vi "Main.vi"() -> ()   [LabVIEW 2021]
uses:
  <vilib>/Instr/_visa.llb/VISA Configure Serial Port (Instr).vi
panel:
  in  "Baud":string(combo)="9600"
  in  "Line Ending":string(combo)="0"
  in  "COM Port":refnum<visa-resource-name>="COM6"
  in  "Enter":bool
  in  "CLEAR":bool
  in  "RESTART COMPORT":bool
  in  "Write to Serial":string
  out "Read from Serial":string
  out "Serial_Thread_state":dbl
  out "Serial_Thread_counter":dbl
  out "Save_Timer_Serial_Thread":dbl
  out "LED_2_state":dbl
  out "LED_2_counter":dbl
  out "Save_Timer_LED_2":dbl
  out "LED_2":bool
  out "Display_1_state":dbl
  out "Display_1_counter":dbl
  out "Save_Timer_Display_1":dbl
  out "LED_1_state":dbl
  out "LED_1_counter":dbl
  out "Save_Timer_LED_1":dbl
  out "LED_1":bool
  in  "Button_1":bool
  in  "Button_2":bool
  in  "CLOSE APP":bool
  out "Display_1":dbl
  # "Press ADD or SUB to add/subtract a value of 1 into the Display_1. Buttons are being monitored while 2 LEDs are\nblinking with different periods. This whole system is executed in multitask process. You may notice that LEDs are\nnot affected nor the buttons are affected to each other. No delay at all."
  # "Note:\nDo not Run the program without Device Connected to the Serial Port.\nIf Error occured because nothing is connected to the comport, just click Continue."
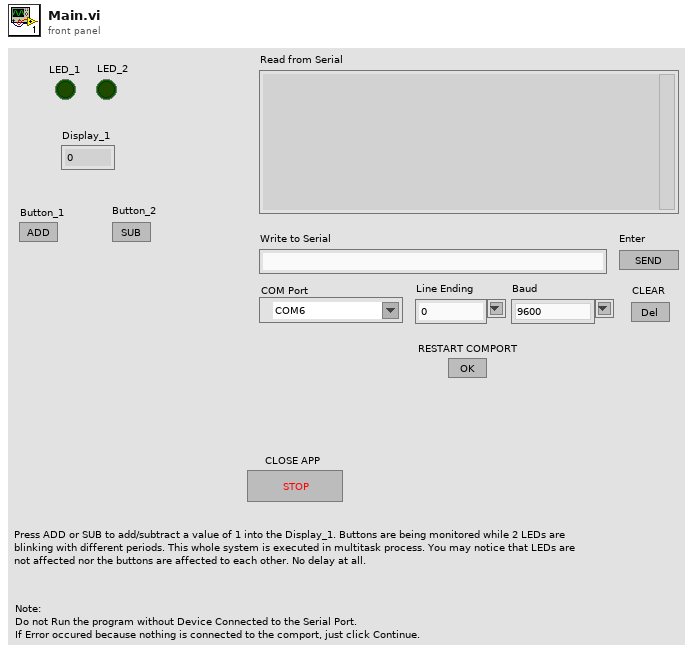
[diagram p1: front panel]
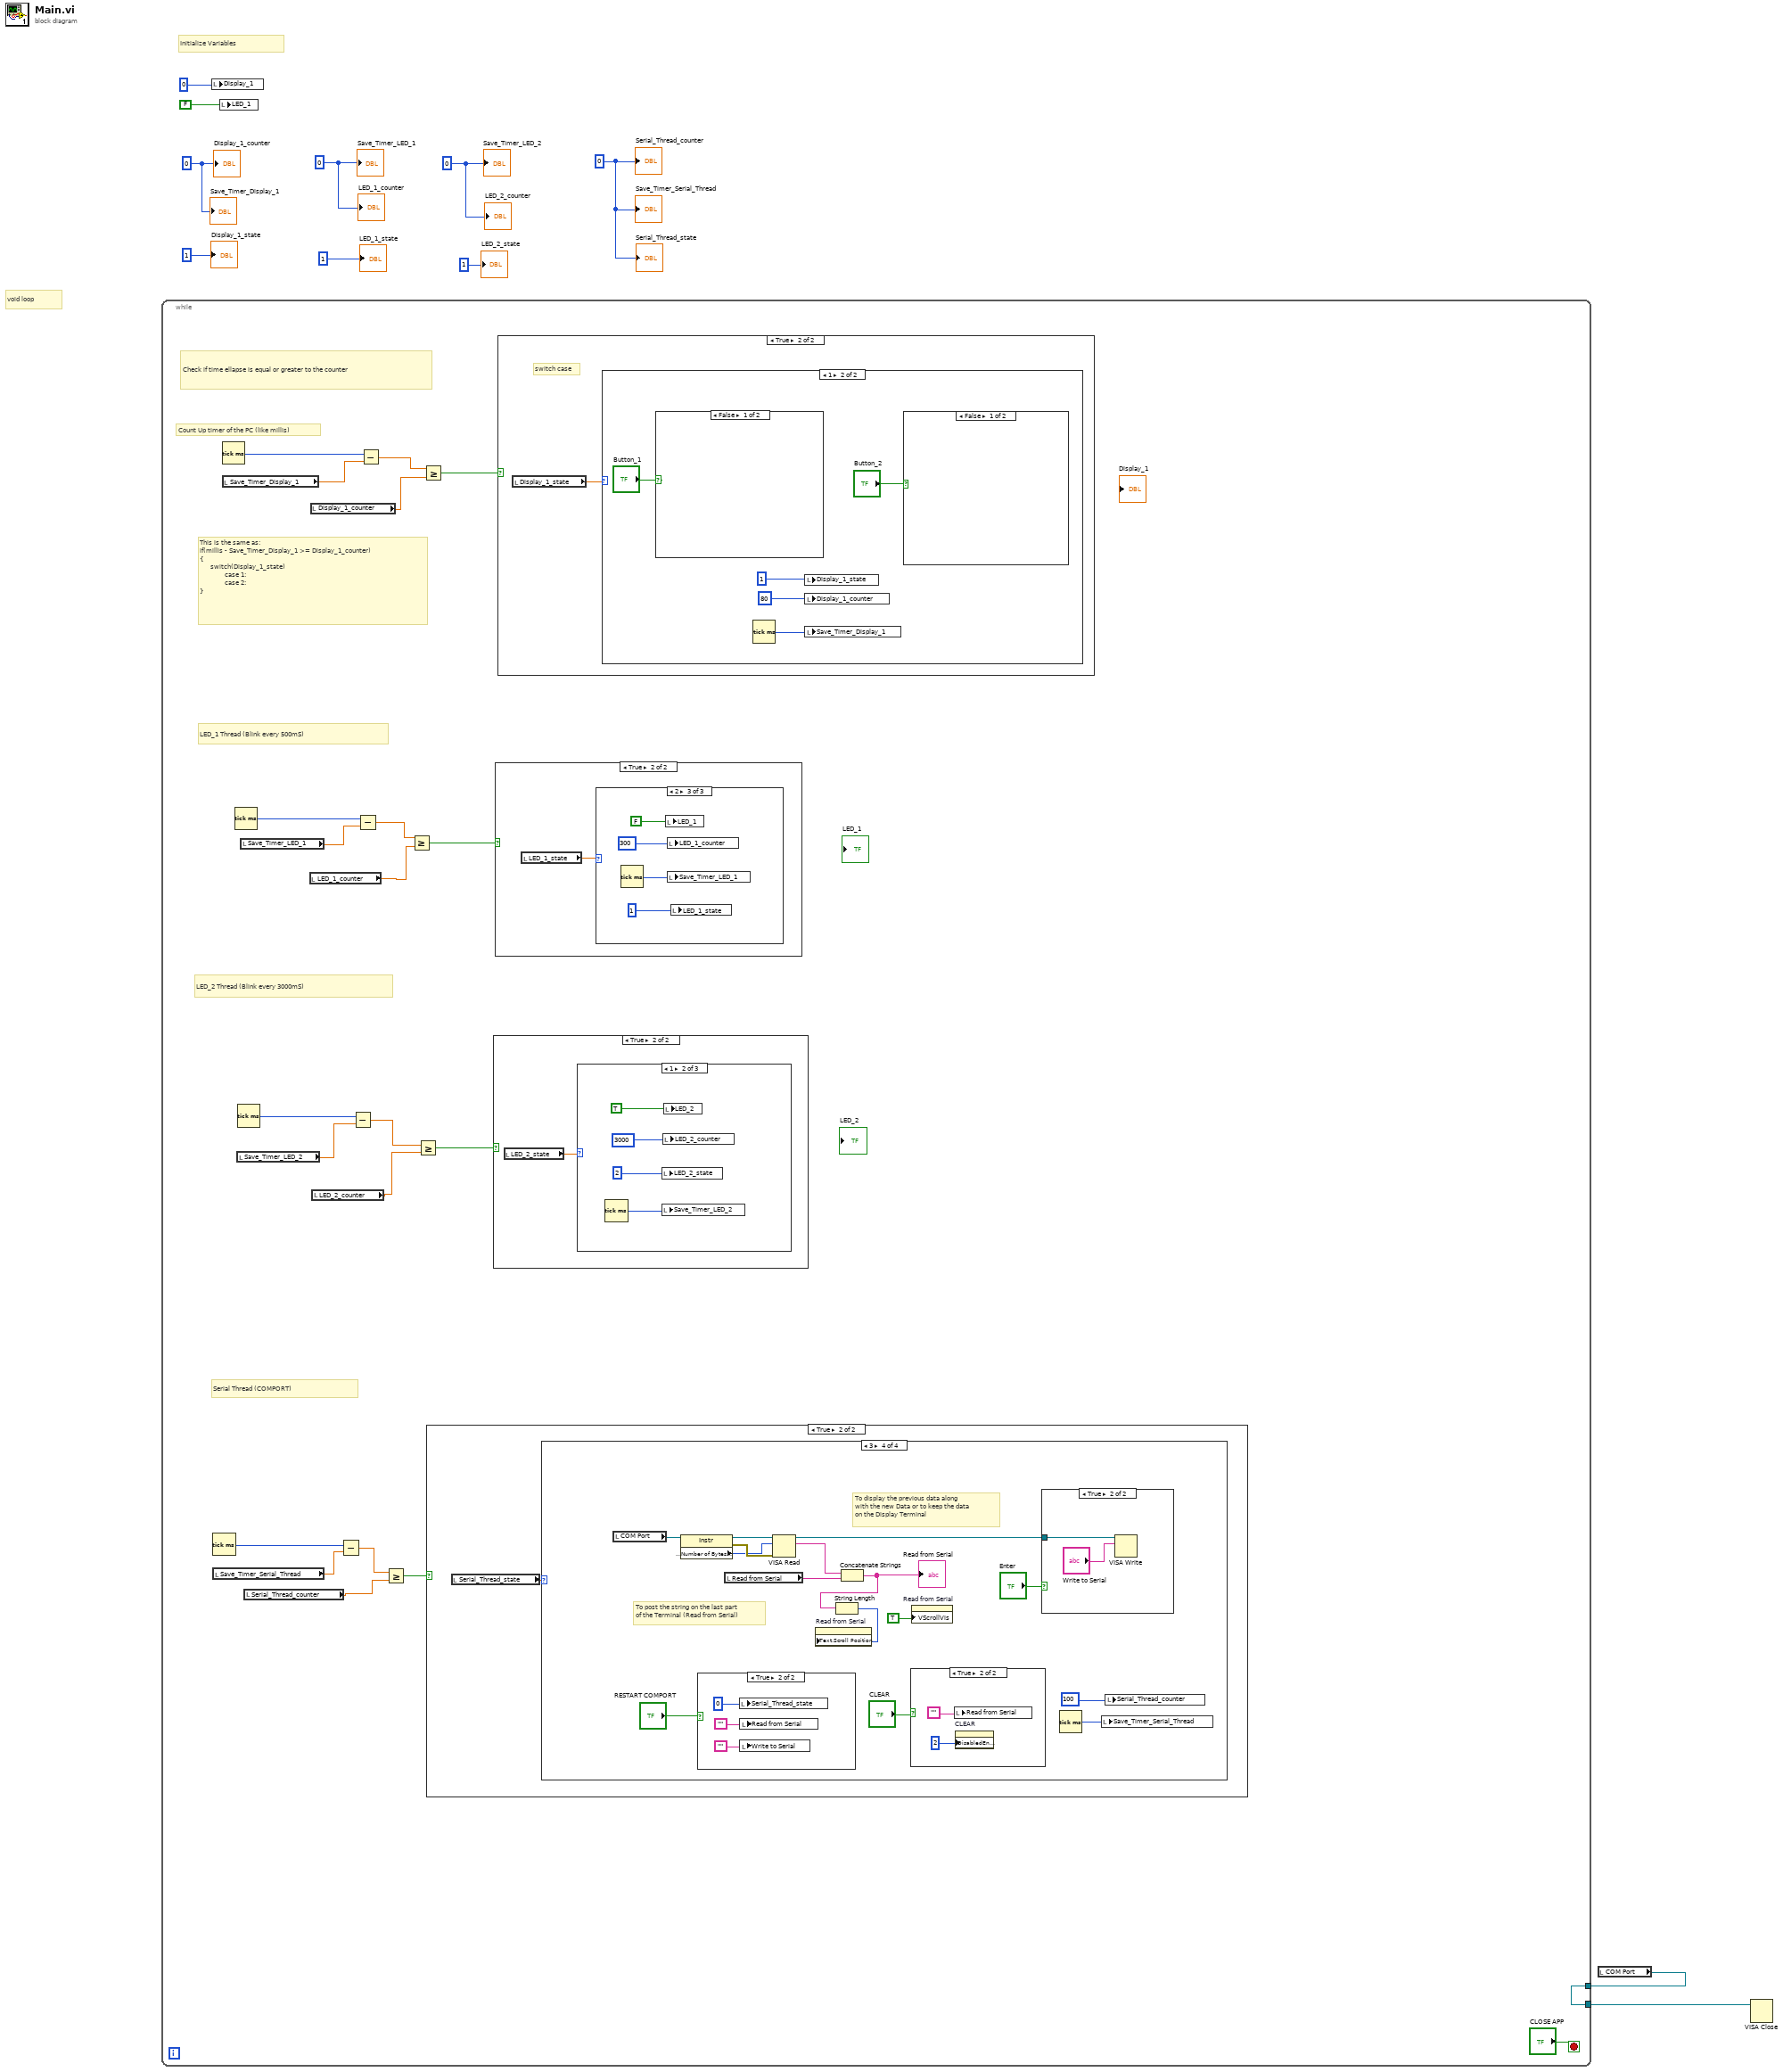
[diagram p0: block diagram]
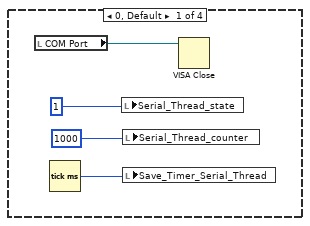
[diagram p3: hidden frame]
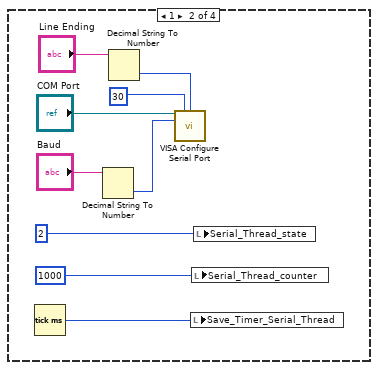
[diagram p4: hidden frame]
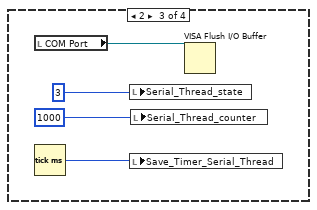
[diagram p5: hidden frame]
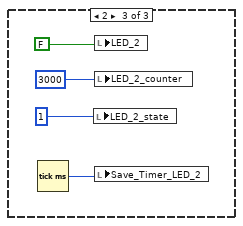
[diagram p11: hidden frame]
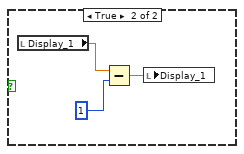
[diagram p14: hidden frame]
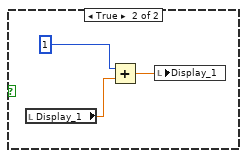
[diagram p15: hidden frame]
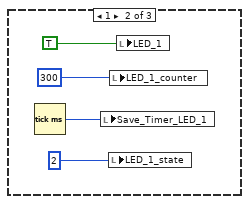
[diagram p18: hidden frame]
diagram:
  w4 = 0
  w2 = 0
  w1 = 0
  w3 = 0
  # "void loop"
  # "Initialize Variables"
  n1 = local write "Display_1"(0) -> ()
  n2 = local write "LED_1"(FALSE) -> ()
  n3 = local read "COM Port"() -> (w5:refnum<visa-resource-name>)
  n4 = while {
    tunnel: [w12] -> w6
    tunnel: w5 -> [w12]
    stop <- "CLOSE APP" stop-if-true
    # "Serial Thread (COMPORT)"
    # "LED_2 Thread (Blink every 3000mS)"
    # "LED_1 Thread (Blink every 500mS)"
    # "This is the same as:\nif(millis - Save_Timer_Display_1 >= Display_1_counter)\n{\n      switch(Display_1_state)\n              case 1:\n              case 2:\n}"
    # "Check if time ellapse is equal or greater to the counter"
    # "Count Up timer of the PC (like millis)"
    n5 = Tick Count (ms)() -> (millisecond timer value=w17:u32)
    n6 = local read "Save_Timer_Serial_Thread"() -> (w16:dbl)
    n7 = Tick Count (ms)() -> (millisecond timer value=w27:u32)
    n8 = local read "Save_Timer_Display_1"() -> (w26:dbl)
    n9 = Tick Count (ms)() -> (millisecond timer value=w32:u32)
    n10 = local read "Save_Timer_LED_2"() -> (w21:dbl)
    n11 = Tick Count (ms)() -> (millisecond timer value=w22:u32)
    n12 = local read "Save_Timer_LED_1"() -> (w31:dbl)
    n13 = local read "Serial_Thread_counter"() -> (w14:dbl)
    n14 = local read "LED_1_counter"() -> (w30:dbl)
    n15 = local read "Display_1_counter"() -> (w24:dbl)
    n16 = local read "LED_2_counter"() -> (w19:dbl)
    n17 = Subtract(x=w17, y=w16) -> (x-y=w15:dbl)
    n18 = Subtract(x=w22, y=w21) -> (x-y=w20:dbl)
    n19 = Subtract(x=w32, y=w31) -> (x-y=w29:dbl)
    n20 = Subtract(x=w27, y=w26) -> (x-y=w25:dbl)
    n21 = Greater Or Equal?(x=w15, y=w14) -> (x >= y?=w13:bool)
    n22 = Greater Or Equal?(x=w29, y=w30) -> (x >= y?=w28:bool)
    n23 = Greater Or Equal?(x=w20, y=w19) -> (x >= y?=w18:bool)
    n24 = Greater Or Equal?(x=w25, y=w24) -> (x >= y?=w23:bool)
    n25 = case shown="True" w13 {
      frame False {
      }
      frame True {
        n26 = local read "Serial_Thread_state"() -> (w34:dbl)
        n27 = case shown="3" w34 {
          frame 0, Default {
            n28 = local read "COM Port"() -> (w38:refnum<visa-resource-name>)
            n29 = Tick Count (ms)() -> (millisecond timer value=w35:u32)
            n30 = local write "Serial_Thread_state"(1) -> ()
            n31 = local write "Serial_Thread_counter"(1000) -> ()
            n32 = local write "Save_Timer_Serial_Thread"(w35) -> ()
            n33 = VISA Close(VISA resource name=w38) -> ()  [unwired: 1 in, 1 out]
          }
          frame 1 {
            n34 = Tick Count (ms)() -> (millisecond timer value=w39:u32)
            n35 = Decimal String To Number(string="Baud") -> (number=w40:i32)  [unwired: 2 in, 1 out]
            n36 = Decimal String To Number(string="Line Ending") -> (number=w43:i32)  [unwired: 2 in, 1 out]
            n37 = call-poly "VISA Configure Serial Port"("VISA resource name"="COM Port", "timeout (10sec)"=30, "termination char\n(0xA = '\\n' = LF)"=w43, "baud rate (9600)"=w40) -> ()  [unwired: 10 in, 2 out]
            n38 = local write "Save_Timer_Serial_Thread"(w39) -> ()
            n39 = local write "Serial_Thread_counter"(1000) -> ()
            n40 = local write "Serial_Thread_state"(2) -> ()
          }
          frame 2 {
            n41 = local read "COM Port"() -> (w51:refnum<visa-resource-name>)
            n42 = Tick Count (ms)() -> (millisecond timer value=w49:u32)
            n43 = local write "Serial_Thread_state"(3) -> ()
            n44 = local write "Save_Timer_Serial_Thread"(w49) -> ()
            n45 = local write "Serial_Thread_counter"(1000) -> ()
            n46 = VISA Flush I/O Buffer(VISA resource name=w51) -> ()  [unwired: 2 in, 2 out]
          }
          frame 3 {
            # "To display the previous data along\nwith the new Data or to keep the data\non the Display Terminal"
            # "To post the string on the last part \nof the Terminal (Read from Serial)"
            n47 = local read "COM Port"() -> (w54:refnum<visa-resource-name>)
            n48 = property class="Instr"(reference=w54) -> (reference out=w63:refnum<visa-resource-name>, error out=w62:errorcluster, "Serial Settings:Number of Bytes at Serial Port"=w61:u32)  [unwired: 1 in]
            n49 = case shown="True" "RESTART COMPORT" {
              frame False {
              }
              frame True {
                n50 = local write "Serial_Thread_state"(0) -> ()
                n51 = local write "Read from Serial"("") -> ()
                n52 = local write "Write to Serial"("") -> ()
              }
            }
            n53 = local read "Read from Serial"() -> (w59:string)
            n54 = VISA Read(VISA resource name=w63, byte count=w61, error in (no error)=w62) -> (VISA resource name out=w55:refnum<visa-resource-name>, read buffer=w60:string)  [unwired: 2 out]
            n55 = Concatenate Strings(w60, w59) -> (w58:string)
            "Read from Serial" <- w58
            n56 = String Length(string=w58) -> (length=w57:i32)
            n57 = property on="Read from Serial" class="Str"("Text.Scroll Position"=w57) -> ()  [unwired: 2 in, 2 out]
            n58 = case shown="True" "CLEAR" {
              frame False {
              }
              frame True {
                n59 = local write "Read from Serial"("") -> ()
                n60 = property on="CLEAR" class="Bool"("DisabledEnum"=2) -> ()  [unwired: 2 in, 2 out]
              }
            }
            n61 = property on="Read from Serial" class="Str"("VScrollVis"=TRUE) -> ()  [unwired: 2 in, 2 out]
            n62 = case shown="True" "Enter" {
              tunnel: w55 -> [_ w73]
              frame False {
              }
              frame True {
                n63 = VISA Write(VISA resource name=w73, write buffer="Write to Serial") -> ()  [unwired: 1 in, 3 out]
              }
            }
            n64 = Tick Count (ms)() -> (millisecond timer value=w64:u32)
            n65 = local write "Save_Timer_Serial_Thread"(w64) -> ()
            n66 = local write "Serial_Thread_counter"(100) -> ()
          }
        }
      }
    }
    n67 = case shown="True" w18 {
      frame False {
      }
      frame True {
        n68 = local read "LED_2_state"() -> (w74:dbl)
        n69 = case shown="1" w74 {
          frame 0, Default {
          }
          frame 1 {
            n70 = Tick Count (ms)() -> (millisecond timer value=w75:u32)
            n71 = local write "LED_2_state"(2) -> ()
            n72 = local write "Save_Timer_LED_2"(w75) -> ()
            n73 = local write "LED_2_counter"(3000) -> ()
            n74 = local write "LED_2"(TRUE) -> ()
          }
          frame 2 {
            n75 = Tick Count (ms)() -> (millisecond timer value=w79:u32)
            n76 = local write "LED_2_state"(1) -> ()
            n77 = local write "LED_2"(FALSE) -> ()
            n78 = local write "LED_2_counter"(3000) -> ()
            n79 = local write "Save_Timer_LED_2"(w79) -> ()
          }
        }
      }
    }
    n80 = case shown="True" w28 {
      frame False {
      }
      frame True {
        n81 = local read "LED_1_state"() -> (w95:dbl)
        n82 = case shown="2" w95 {
          frame 0, Default {
          }
          frame 1 {
            n83 = Tick Count (ms)() -> (millisecond timer value=w99:u32)
            n84 = local write "Save_Timer_LED_1"(w99) -> ()
            n85 = local write "LED_1_state"(2) -> ()
            n86 = local write "LED_1_counter"(300) -> ()
            n87 = local write "LED_1"(TRUE) -> ()
          }
          frame 2 {
            n88 = Tick Count (ms)() -> (millisecond timer value=w101:u32)
            n89 = local write "LED_1"(FALSE) -> ()
            n90 = local write "LED_1_counter"(300) -> ()
            n91 = local write "Save_Timer_LED_1"(w101) -> ()
            n92 = local write "LED_1_state"(1) -> ()
          }
        }
      }
    }
    n93 = case shown="True" w23 {
      frame False {
      }
      frame True {
        # "switch case"
        n94 = local read "Display_1_state"() -> (w83:dbl)
        n95 = case shown="1" w83 {
          frame 0, Default {
          }
          frame 1 {
            n96 = case shown="False" "Button_1" {
              frame False {
              }
              frame True {
                n97 = local read "Display_1"() -> (w93:dbl)
                n98 = Add(x=1, y=w93) -> (x+y=w92:dbl)
                n99 = local write "Display_1"(w92) -> ()
              }
            }
            n100 = Tick Count (ms)() -> (millisecond timer value=w84:u32)
            n101 = local write "Display_1_state"(1) -> ()
            n102 = local write "Display_1_counter"(80) -> ()
            n103 = local write "Save_Timer_Display_1"(w84) -> ()
            n104 = case shown="False" "Button_2" {
              frame False {
              }
              frame True {
                n105 = local read "Display_1"() -> (w91:dbl)
                n106 = Subtract(x=w91, y=1) -> (x-y=w89:dbl)
                n107 = local write "Display_1"(w89) -> ()
              }
            }
          }
        }
      }
    }
  }
  n108 = VISA Close(VISA resource name=w6) -> ()  [unwired: 1 in, 1 out]
  "Save_Timer_LED_1" <- w3
  "LED_1_counter" <- w3
  "LED_1_state" <- 1
  "Save_Timer_Display_1" <- w1
  "Display_1_counter" <- w1
  "Display_1_state" <- 1
  "LED_2_counter" <- w2
  "Save_Timer_LED_2" <- w2
  "LED_2_state" <- 1
  "Save_Timer_Serial_Thread" <- w4
  "Serial_Thread_counter" <- w4
  "Serial_Thread_state" <- w4
